vi "TCP.IP_Python for data.vi"(8 "error in (no error)":errorcluster, 10 "loop 1":i32, 11 "Refnum in":refnum<k35>) -> (0 "error out":errorcluster, 2 "Array":dbl[](array[numeric]), 3 "Refnum out":refnum<k35>)   [LabVIEW 2021]
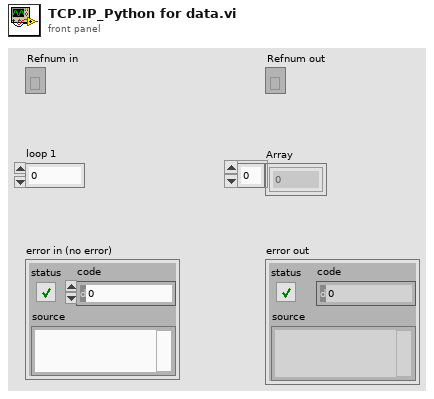
[diagram p1: front panel]
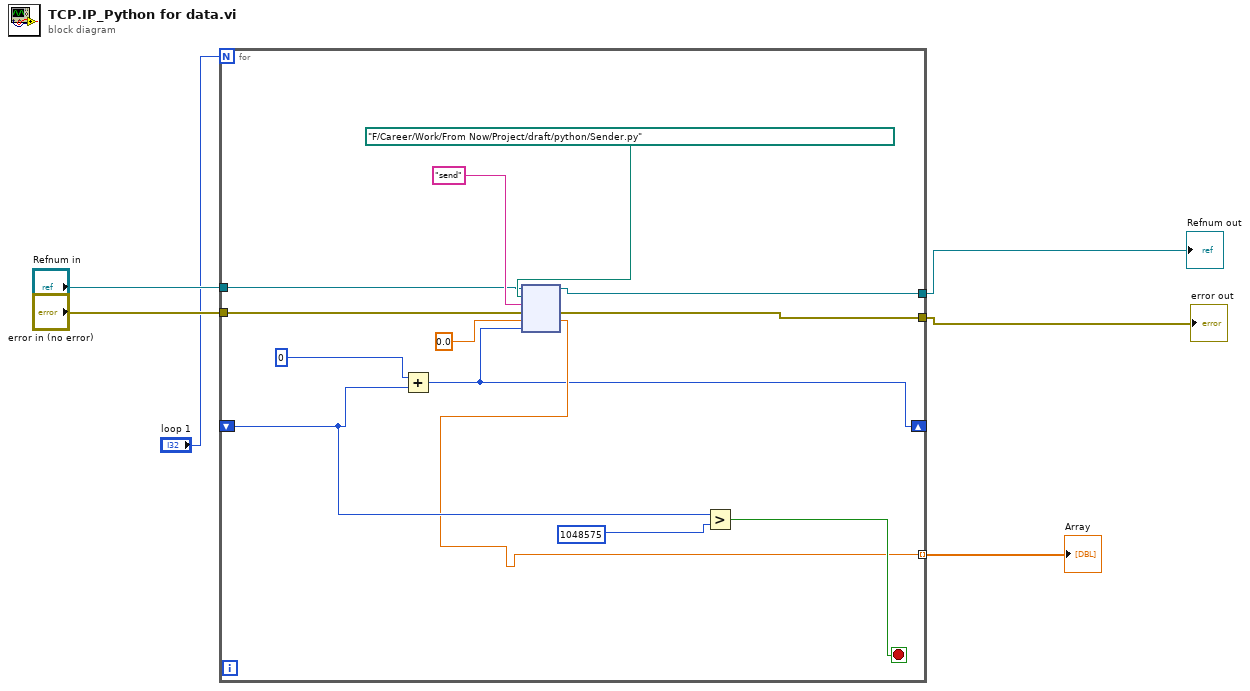
[diagram p0: block diagram]
diagram:
  n1 = for {
    N: "loop 1" -> [_]
    tunnel: [w11] -> w2 mode=indexing
    tunnel: [w17] -> w5
    tunnel: [w16] -> w6
    tunnel: "Refnum in" -> [w15]
    tunnel: "error in (no error)" -> [w14]
    shift-right: [w10] -> _
    shift-left: _ -> [w13]
    stop <- w12 stop-if-true
    n2 = Add(x=0, y=w13) -> (x+y=w10:i32)
    n3 = node(w15, path "F:/Career/Work/From Now/Project/draft/python/Sender.py" ("module path"), "send" ("function name"), w14, 0.0, w10) -> (w17:refnum<k35>, w16:errorcluster, w11:dbl)  [unwired: 1 in, 2 out]
    n4 = Greater?(x=w13, y=1048575) -> (0:w12:bool)
  }
  "error out" <- w6
  "Refnum out" <- w5
  "Array" <- w2
